vi "WaveformTUA(SubVI).vi"(8 "error in (no error)":errorcluster, 10 "WF in":dbl[][](array[numeric]), 11 "new reference":refnum<k24>) -> (0 "error out":errorcluster, 2 "WF out":dbl[](array[numeric]), 3 "reference out":refnum<k24>)   [LabVIEW 2024]
uses:
  C:/Users/MarcuLab/Documents/GitHub/NetDeconForLV/Source/DotNETAssembly1.0.3/output/build/LaguerreDeconRTNative.dll
  Documents/GitHub/NetDeconForLV/Source/DotNETAssembly1.0.3/output/build/LaguerreDeconRTNative.dll
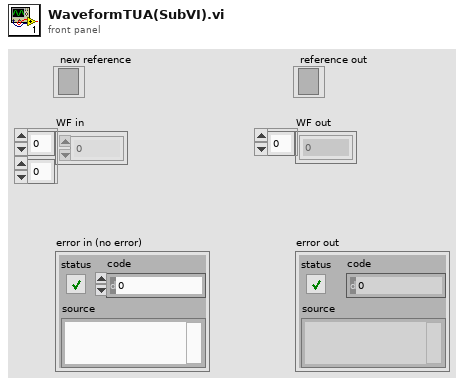
[diagram p1: front panel]
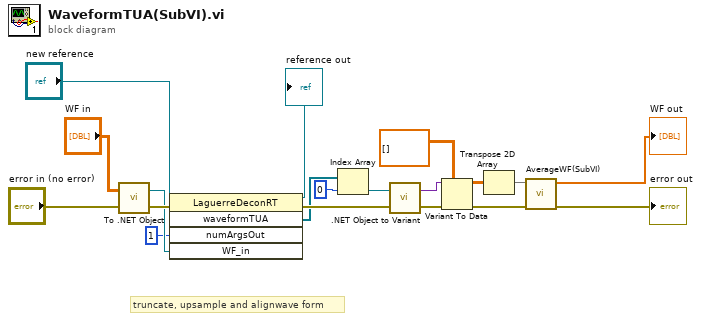
[diagram p0: block diagram]
diagram:
  # "truncate, upsample and alignwave form"
  n1 = call <vilib>:"To .NET Object.vi"("error in (no error)"="error in (no error)", "anything"="WF in") -> ("error out"=w6:errorcluster, ".NET object"=w5:refnum<k24>)
  n2 = invoke class="LaguerreDeconRT" method="waveformTUA"(reference="new reference", error in=w6, "numArgsOut"=1, "WF_in"=w5) -> (reference out=→"reference out":refnum<k24>, error out=w13:errorcluster, "waveformTUA"=w12:refnum<k24>[])  [unwired: 1 in, 2 out]
  n3 = Index Array(array=w12, index=0) -> (element=w8:refnum<k24>)
  n4 = call <vilib>:".NET Object to Variant.vi"("error in (no error)"=w13, ".NET object"=w8) -> ("error out"=w10:errorcluster, "variant"=w11:variant)
  n5 = Variant To Data(error in=w10, type=dbl[][] [], Variant=w11) -> (data=w9:dbl[][], error out=w16:errorcluster)
  n6 = Transpose 2D Array(2D array=w9) -> (transposed array=w15:dbl[][])
  n7 = call "AverageWF(SubVI).vi"("error in (no error)"=w16, "Array in"=w15) -> ("error out"=→"error out":errorcluster, "Array out"=→"WF out":dbl[])  [unwired: 8 in]
